vi "Acquisition_b.vi"() -> (4 "Acquired_Data":dbl(graph))   [LabVIEW 2021]
doc: "This VI acquire data that were generated be the Generator VI.\nTransfer of thet data happens under Simple LV2."
uses:
  Type_Def/Operation_Simple_LV2.ctl
panel:
  out "Error_Out":errorcluster
  in  "Error_In":errorcluster
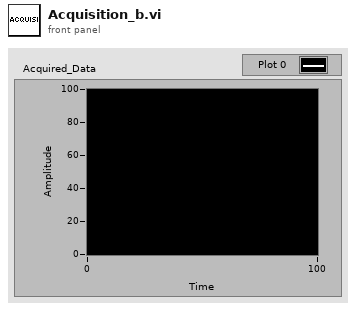
[diagram p1: front panel]
types:
  T1 = typedef "Operation_Simple_LV2.ctl" = u16
  T2 = enum16{"Left Button", "Center Button", "Right Button", "Window Close"}
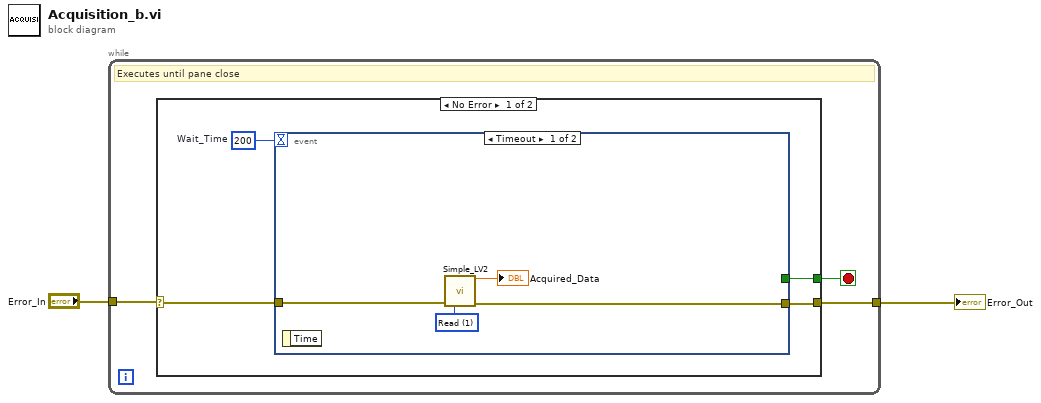
[diagram p0: block diagram]
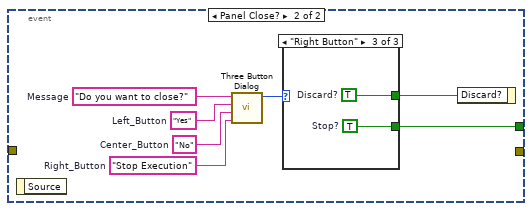
[diagram p2: hidden frame]
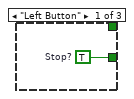
[diagram p3: hidden frame]
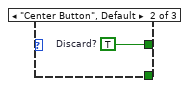
[diagram p4: hidden frame]
diagram:
  n1 = while {
    tunnel: "Error_In" -> [w4]
    tunnel: [w3] -> w1
    stop <- w5 stop-if-true
    # "Executes until pane close"
    n2 = case shown="No Error" w4 {
      selector: w4 -> [w7 w25]
      tunnel: [w8 _] -> w5
      tunnel: [w6 w25] -> w3
      frame No Error {
        w9 = 200  # Wait_Time
        n3 = event shown="[0] Timeout" {
          selector: _ -> [_ _]
          dyn-events: _ -> [_ _]
          timeout: w9 -> [_ _]
          tunnel: [_ w14] -> w8
          tunnel: w7 -> [w11 _]
          tunnel: [w10 _] -> w6
          event Timeout {
            w13 = T1 1 items=["Write", "Read"] ("Ring")
            n4 = event-data() -> ()  [unwired: 1 in, 1 out]
            n5 = call "Simple_LV2.vi"("Error_In"=w11, "Operation"=w13) -> ("Data_Out"=→"Acquired_Data":dbl, "Error_Out"=w10:errorcluster)  [unwired: 12 in]
          }
          event Panel Close? {
            w17 = "Stop Execution"  # Right_Button
            w18 = "No"  # Center_Button
            w19 = "Yes"  # Left_Button
            w20 = "Do you want to close?"  # Message
            n6 = event-data() -> ()  [unwired: 1 in, 1 out]
            n7 = call <vilib>:"Three Button Dialog.vi"("Right Button Text (\"Cancel\")"=w17, "Center Button Text (\"No\")"=w18, "Left Button Text (\"Yes\")"=w19, "message"=w20) -> ("Which Button?"=w16:T2)  [unwired: 7 in]
            n8 = case shown="\"Right Button\"" w16 {
              tunnel: [_ w22 w23] -> w15
              tunnel: [w21 _ w24] -> w14
              frame "Left Button" {
                w21 = TRUE  # Stop?
              }
              frame "Center Button", Default {
                w22 = TRUE  # Discard?
              }
              frame "Right Button" {
                w23 = TRUE  # Discard?
                w24 = TRUE  # Stop?
              }
            }
            n9 = event-data("Discard?"=w15) -> ()  [unwired: 1 in, 1 out]
          }
        }
      }
      frame Error {
      }
    }
  }
  "Error_Out" <- w1
